vi "Motor.vi"(6 "Speed":u16, 7 "枚举":T1(ring), 8 "Pulse":i32, 9 "Move Type":u16(ring)=3 items=["Relative", "absolutely", "TSL", "Go Home", "Reserve 1", "Reserve 2", "Clean Alarm", "Reserve 3", "Decelerate_Stop", "Emergency stop", "Reserve 4", "Jog+", "Jog-"], 10 "Servo ON/OFF":bool=TRUE, 11 "VISA resource name":refnum<visa-resource-name>) -> (1 "Position":u32, 2 "Motion Down":bool, 3 "VISA resource name out":refnum<visa-resource-name>)   [LabVIEW 2017]
uses:
  NI Modbus.llb/MB Serial Master Query Write Single Register (poly).vi
  NI Modbus.llb/MB Serial Master Query Read Holding Registers (poly).vi
  NI Modbus.llb/MB Serial Master Query Write Multiple Registers (poly).vi
panel:
  out "Alarm":bool
  in  "error in":errorcluster
  out "Servo ON":bool
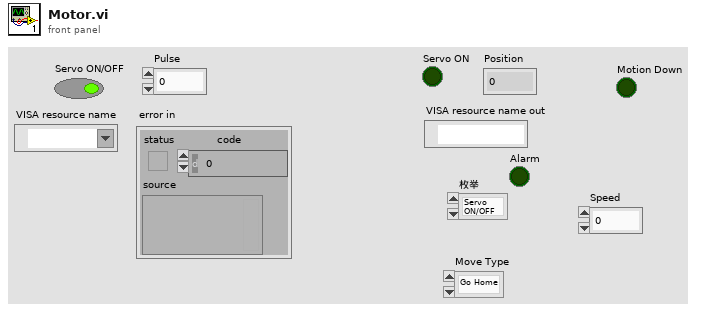
[diagram p1: front panel]
types:
  T1 = enum16{"Servo ON/OFF", "Move Type", "Action Status", "Location", "Motor Status", "Move Pulse", "Move Speed"}
  T2 = cluster{"Mode":enum16{"RTU", "ASCII"}, "Slave Address":u8}
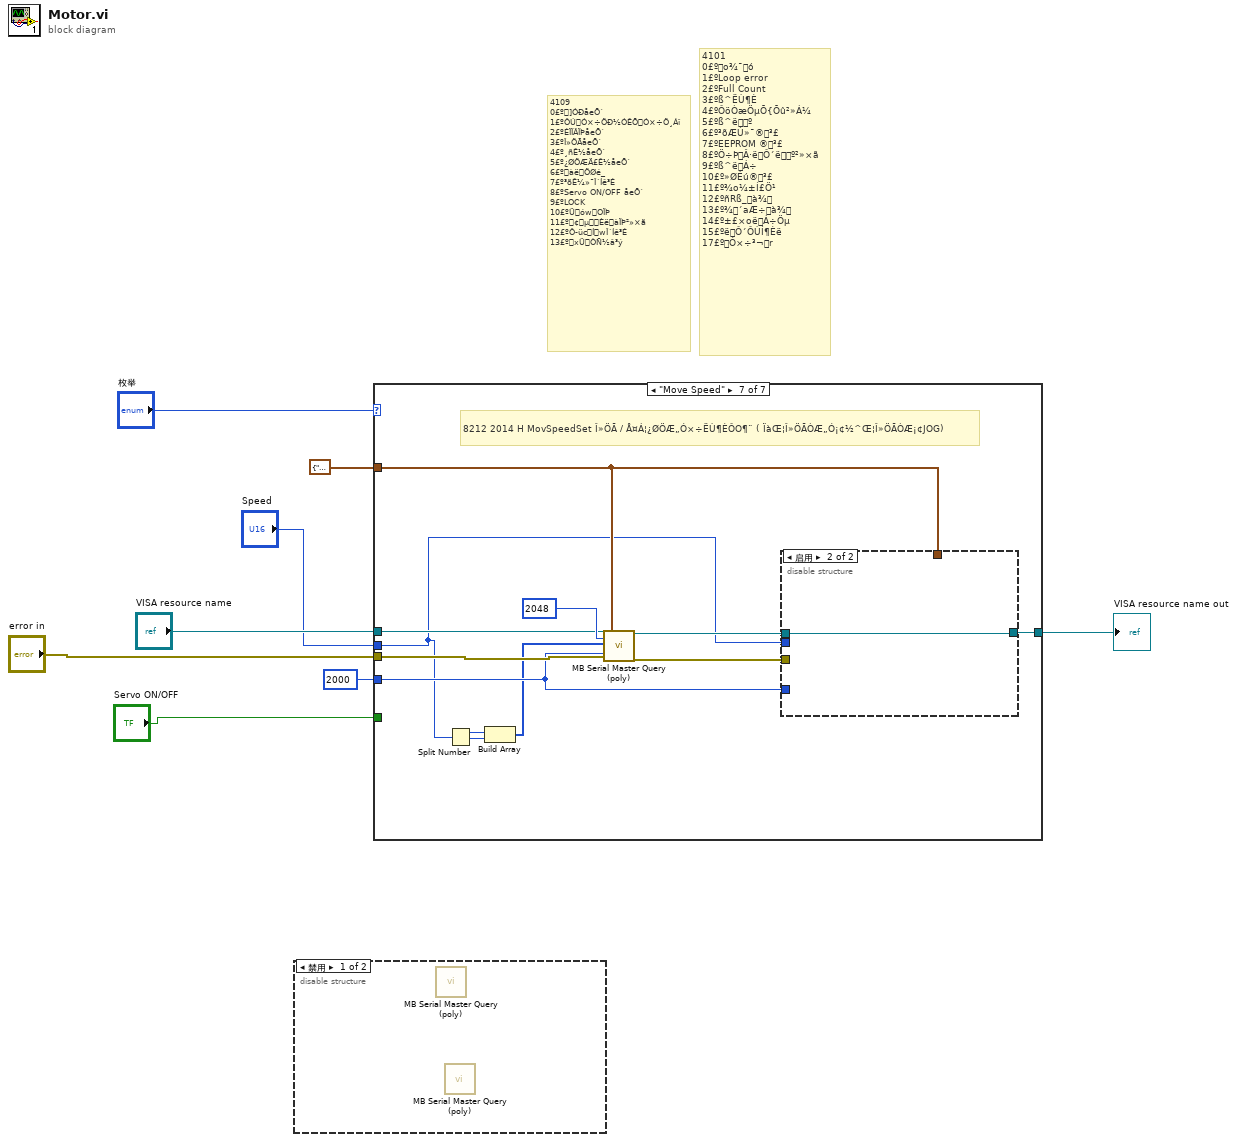
[diagram p0: block diagram]
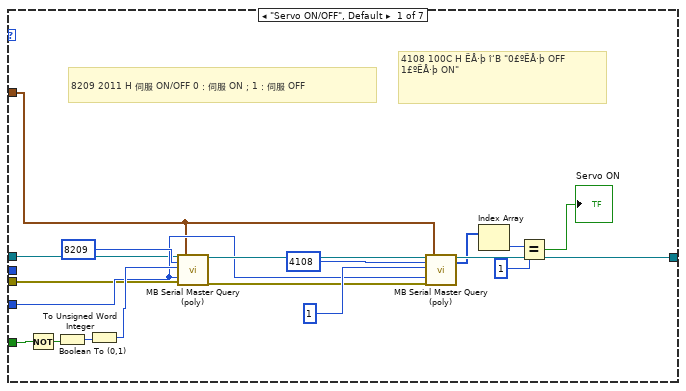
[diagram p2: hidden frame]
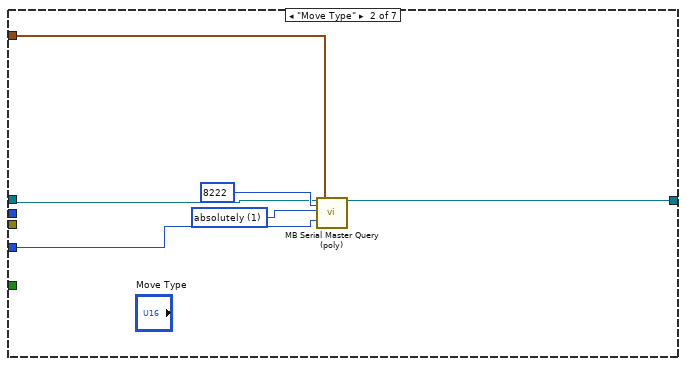
[diagram p3: hidden frame]
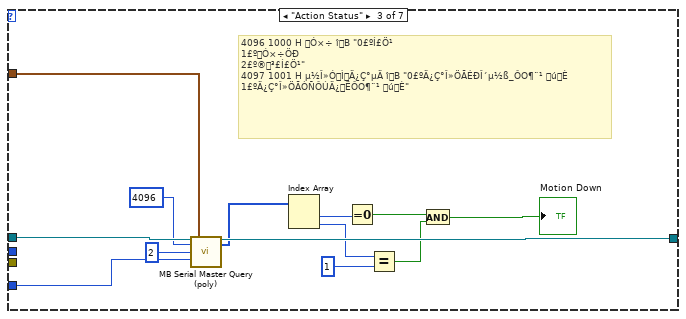
[diagram p4: hidden frame]
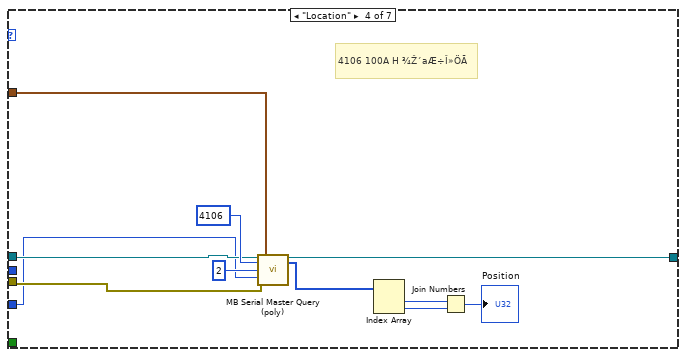
[diagram p5: hidden frame]
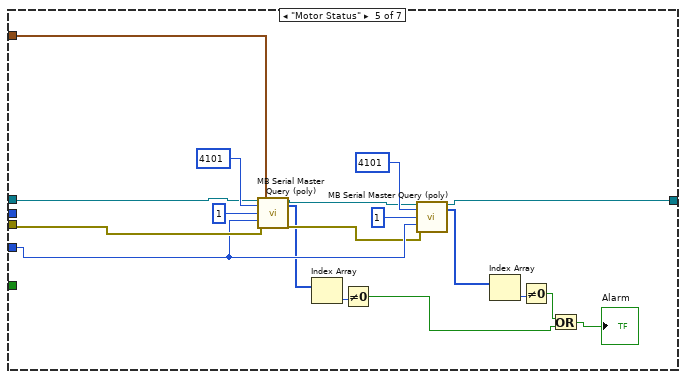
[diagram p6: hidden frame]
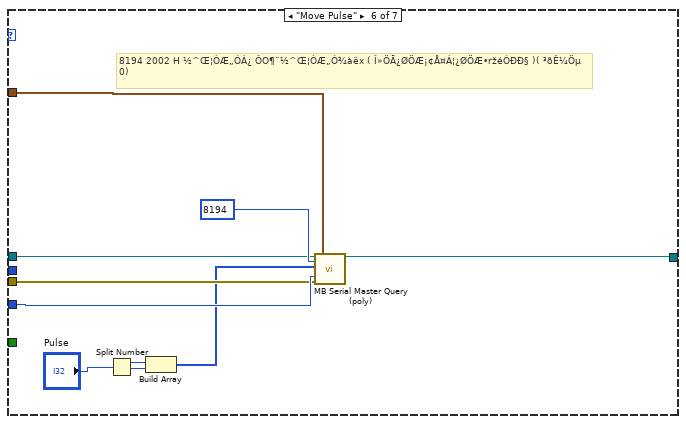
[diagram p7: hidden frame]
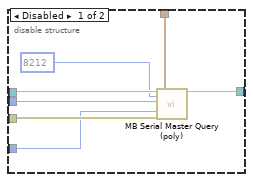
[diagram p8: hidden frame]
diagram:
  # "4101\n0£ºo¾¯ó\n1£ºLoop error\n2£ºFull Count\n3£ºß^ËÙ¶È\n4£ºÔöÒæÖµÕ{Õû²»Á¼\n5£ºß^ëº\n6£º³õÆÚ»¯®³£\n7£ºEEPROM ®³£\n8£ºÖ÷ÞÂ·ëÔ´ëº²»×ã\n9£ºß^ëÁ÷\n10£º»ØÉú®³£\n11£º¾o¼±Í£Ö¹\n12£ºñRß_à¾\n13£º¾´aÆ÷à¾\n14£º±£×oëÁ÷Öµ\n15£ºëÔ´ÔÙÍ¶Èë\n17£ºÓ×÷³¬r"
  # "4109\n0£º]ÓÐåeÕ`\n1£ºÔÚÓ×÷ÖÐ½ÓÊÕÓ×÷Ö¸Áî\n2£ºÉÏÏÂÏÞåeÕ`\n3£ºÎ»ÖÃåeÕ`\n4£º¸ñÊ½åeÕ`\n5£º¿ØÖÆÄ£Ê½åeÕ`\n6£ºàëÖØé_\n7£º³õÊ¼»¯Î´Íê³É\n8£ºServo ON/OFF åeÕ`\n9£ºLOCK\n10£ºÜówOÏÞ\n11£º¢µÈëàÏÞ²»×ã\n12£ºÔ­ücÍwÎ´Íê³É\n13£ºxÜÒÑ½â³ý"
  n1 = disable-structure shown="禁用" {
    frame Disabled {
      n2 = call-poly "MB Serial Master Query (poly).vi"() -> ()  [unwired: 17 in, 3 out]
      n3 = call-poly "MB Serial Master Query (poly).vi"() -> ()  [unwired: 17 in, 3 out]
    }
    frame Enabled {
    }
  }
  n4 = case shown="\"Move Speed\"" "枚举" {
    tunnel: [w19 w30 w44 w47 w60 w79 w92] -> w7
    tunnel: u32 2000 ("Timeout") -> [w13 w31 w43 w52 w66 w81 w89]
    tunnel: T2 {"Mode"=enum."RTU", "Slave Address"=1} ("Serial Parameters") -> [w12 w29 w33 w46 w70 w82 w91]
    tunnel: "VISA resource name" -> [w11 w28 w45 w54 w72 w83 w95]
    tunnel: "error in" -> [w10 _ _ w53 w71 w80 w94]
    tunnel: "Speed" -> [_ _ _ _ _ _ w85]
    tunnel: "Servo ON/OFF" -> [w9 _ _ _ _ _ _]
    frame "Servo ON/OFF", Default {
      # "4108\t100C H\tËÅ·þ î‘B\t\"0£ºËÅ·þ OFF\n1£ºËÅ·þ ON\""
      # "8209\t2011 H\t伺服 ON/OFF\t0：伺服 ON；1：伺服 OFF"
      n5 = Not(x=w9) -> (.not. x?=w22:bool)
      n6 = Boolean To (0,1)(Boolean=w22) -> (0, 1=w21:i16)
      n7 = To Unsigned Word Integer(number=w21) -> (unsigned 16bit integer=w20:u16)
      n8 = call-poly "MB Serial Master Query (poly).vi"("VISA resource name"=w11, "Address"=u16 8209, "Holding Register"=w20, "Timeout"=w13, "error in"=w10, "Serial Parameters"=w12) -> ("VISA resource name out"=w23:refnum<visa-resource-name>, "error out"=w18:errorcluster)  [unwired: 11 in, 1 out]
      n9 = call-poly "MB Serial Master Query (poly).vi"("VISA resource name"=w23, "Starting Address"=u16 4108, "Quantity"=u16 1, "Timeout"=w13, "error in"=w18, "Serial Parameters"=w12) -> ("VISA resource name out"=w19:refnum<visa-resource-name>, "Holding Registers"=w17:u16[])  [unwired: 10 in, 2 out]
      n10 = Index Array(array=w17) -> (element=w16:u16)  [unwired: 1 in]
      n11 = Equal?(x=w16, y=u16 1) -> (x = y?=→"Servo ON":bool)
    }
    frame "Move Type" {
      w27 = u16 1 items=["Relative", "absolutely", "TSL", "Go Home", "Reserve 1", "Reserve 2", "Clean Alarm", "Reserve 3", "Decelerate_Stop", "Emergency stop", "Reserve 4", "Jog+", "Jog-"] ("Move Type 2")
      n12 = call-poly "MB Serial Master Query (poly).vi"("VISA resource name"=w28, "Address"=u16 8222, "Holding Register"=w27, "Timeout"=w31, "Serial Parameters"=w29) -> ("VISA resource name out"=w30:refnum<visa-resource-name>)  [unwired: 12 in, 2 out]
    }
    frame "Action Status" {
      # "4096\t1000 H\tÓ×÷ îB\t\"0£ºÍ£Ö¹\n1£ºÓ×÷ÖÐ\n2£º®³£Í£Ö¹\"\n4097\t1001 H\tµ½Î»ÓÌÄ¿Ç°µÄ îB\t\"0£ºÄ¿Ç°Î»ÖÃÉÐÎ´µ½ß_ÔO¶¨¹ úÈ\n1£ºÄ¿Ç°Î»ÖÃÒÑÔÚÄ¿ËÔO¶¨¹ úÈ\""
      n13 = call-poly "MB Serial Master Query (poly).vi"("VISA resource name"=w45, "Starting Address"=u16 4096, "Quantity"=u16 2, "Timeout"=w43, "Serial Parameters"=w33) -> ("VISA resource name out"=w44:refnum<visa-resource-name>, "Holding Registers"=w40:u16[])  [unwired: 11 in, 2 out]
      n14 = Index Array(array=w40) -> (element #1=w39:u16, element #2=w38:u16)  [unwired: 2 in]
      n15 = Equal To 0?(x=w39) -> (x = 0?=w36:bool)
      n16 = Equal?(x=w38, y=u16 1) -> (x = y?=w35:bool)
      n17 = And(x=w36, y=w35) -> (x .and. y?=→"Motion Down":bool)
    }
    frame "Location" {
      # "4106\t100A H\t¾Ž´aÆ÷Î»ÖÃ"
      n18 = call-poly "MB Serial Master Query (poly).vi"("VISA resource name"=w54, "Starting Address"=u16 4106, "Quantity"=u16 2, "Timeout"=w52, "error in"=w53, "Serial Parameters"=w46) -> ("VISA resource name out"=w47:refnum<visa-resource-name>, "Holding Registers"=w51:u16[])  [unwired: 10 in, 2 out]
      n19 = Index Array(array=w51) -> (element #1=w50:u16, element #2=w49:u16)  [unwired: 2 in]
      n20 = Join Numbers(hi=w50, lo=w49) -> ((hi.lo)=→"Position":u32)
    }
    frame "Motor Status" {
      n21 = call-poly "MB Serial Master Query (poly).vi"("VISA resource name"=w72, "Starting Address"=u16 4101, "Quantity"=u16 1, "Timeout"=w66, "error in"=w71, "Serial Parameters"=w70) -> ("VISA resource name out"=w67:refnum<visa-resource-name>, "Holding Registers"=w64:u16[], "error out"=w65:errorcluster)  [unwired: 10 in, 1 out]
      n22 = Index Array(array=w64) -> (element=w63:u16)  [unwired: 1 in]
      n23 = Not Equal To 0?(x=w63) -> (x != 0?=w58:bool)
      n24 = call-poly "MB Serial Master Query (poly).vi"("VISA resource name"=w67, "Starting Address"=u16 4101, "Quantity"=u16 1, "Timeout"=w66, "error in"=w65) -> ("VISA resource name out"=w60:refnum<visa-resource-name>, "Holding Registers"=w61:u16[])  [unwired: 11 in, 2 out]
      n25 = Index Array(array=w61) -> (element=w62:u16)  [unwired: 1 in]
      n26 = Not Equal To 0?(x=w62) -> (x != 0?=w59:bool)
      n27 = Or(x=w59, y=w58) -> (x .or. y?=→"Alarm":bool)
    }
    frame "Move Pulse" {
      # "8194\t2002 H\t½^Œ¦ÒÆ„ÓÁ¿\tÔO¶¨½^Œ¦ÒÆ„Ó¾àëx ( Î»ÖÃ¿ØÖÆ¡¢Å¤Á¦¿ØÖÆ•ržéÓÐÐ§ )( ³õÊ¼Öµ 0)"
      n28 = Split Number(x="Pulse") -> (hi(x)=w78:u16, lo(x)=w77:u16)
      n29 = Build Array(w78, w77) -> (w75:u16[])
      n30 = call-poly "MB Serial Master Query (poly).vi"("VISA resource name"=w83, "Starting Address"=u16 8194 ("Address"), "Registers"=w75, "Timeout"=w81, "error in"=w80, "Serial Parameters"=w82) -> ("VISA resource name out"=w79:refnum<visa-resource-name>)  [unwired: 11 in, 2 out]
    }
    frame "Move Speed" {
      # "8212\t2014 H\tMovSpeedSet\tÎ»ÖÃ / Å¤Á¦¿ØÖÆ„Ó×÷ËÙ¶ÈÔO¶¨ ( ÏàŒ¦Î»ÖÃÒÆ„Ó¡¢½^Œ¦Î»ÖÃÒÆ¡¢JOG)"
      n31 = Split Number(x=w85) -> (hi(x)=w88:u8, lo(x)=w87:u8)
      n32 = Build Array(w88, w87) -> (w86:u8[])
      n33 = call-poly "MB Serial Master Query (poly).vi"("VISA resource name"=w95, "Starting Address"=u16 2048 ("Address"), "Registers"=w86, "Timeout"=w89, "error in"=w94, "Serial Parameters"=w91) -> ("VISA resource name out"=w93:refnum<visa-resource-name>, "error out"=w90:errorcluster)  [unwired: 11 in, 1 out]
      n34 = disable-structure shown="启用" {
        disable-tunnel: w93 -> [w103 w104]
        disable-tunnel: [w102 w104] -> w92
        disable-tunnel: w91 -> [w101 _]
        disable-tunnel: w90 -> [w100 _]
        disable-tunnel: w89 -> [w99 _]
        disable-tunnel: w85 -> [w97 _]
        frame Disabled {
          n35 = call-poly "MB Serial Master Query (poly).vi"("VISA resource name"=w103, "Address"=u16 8212, "Holding Register"=w97, "Timeout"=w99, "error in"=w100, "Serial Parameters"=w101) -> ("VISA resource name out"=w102:refnum<visa-resource-name>)  [unwired: 11 in, 2 out]
        }
        frame Enabled {
        }
      }
    }
  }
  "VISA resource name out" <- w7
